vi "GetDescription.vi"(8 "error in (no error)":errorcluster caption="错误输入（无错误）", 11 "Soy 输入":refnum<class "Soy.lvclass">) -> (0 "error out":errorcluster caption="错误输出", 2 "Description":string, 3 "Soy 输出":refnum<class "Soy.lvclass">)   [LabVIEW 2016, in "Soy.lvclass"]
uses:
  Soy.lvclass
  Soy.lvclass/Soy.ctl
  CondimentDecorator.lvclass
  Beverage.lvclass
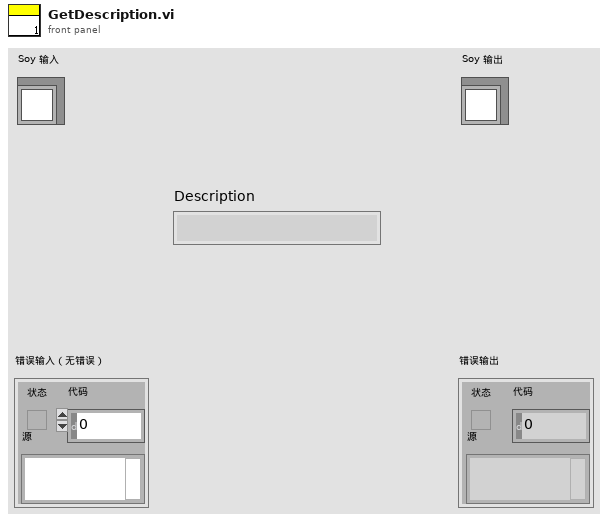
[diagram p1: front panel]
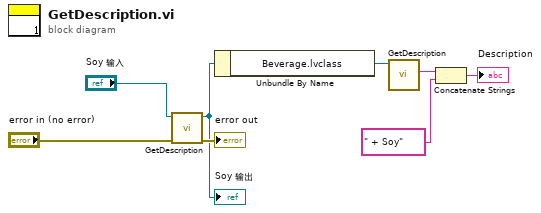
[diagram p0: block diagram]
diagram:
  n1 = call-parent "GetDescription.vi"("error in (no error)"="error in (no error)", "CondimentDecorator 输入"="Soy 输入") -> ("error out"=→"error out":errorcluster, "CondimentDecorator 输出"=w5:refnum<class "Soy.lvclass">)  [unwired: 7 in, 1 out]
  "Soy 输出" <- w5
  n2 = Unbundle By Name(w5) -> ("Beverage.lvclass"=w4:refnum<class "Beverage.lvclass">)
  n3 = call-dynamic "GetDescription.vi"("Beverage 输入"=w4) -> ("Description"=w3:string)  [unwired: 8 in, 2 out]
  n4 = Concatenate Strings(w3, " + Soy" ("字符串")) -> (→"Description":string)
